vi "Detect Modules.vi"(8 "error in":errorcluster, 9 "Chassis in":refnum<class "Chassis.lvclass">, 10 "Controller in":refnum<class "Controller.lvclass">, 11 "Device in":refnum<class "SysCfg Device.lvclass">) -> (0 "error out":errorcluster, 1 "Chassis out":refnum<class "Chassis.lvclass">, 2 "Controller out":refnum<class "Controller.lvclass">, 3 "Device out":refnum<class "SysCfg Device.lvclass">)   [LabVIEW 2015, in "SMI.lvlib" / "Chassis.lvclass"]
uses:
  Chassis.lvclass
  SysCfg Device/SysCfg Device.lvclass
  Controller/Controller.lvclass
  Device/Device.lvclass/Device.ctl
  Chassis.lvclass/Chassis.ctl
  Module/Module.lvclass
  Device/Accessor Methods/Read Product Name.vi
  <vilib>/FPGAPlugInAG/Dynamic/niLvFpga_Close_Dynamic.vi
  <vilib>/regexp/Match Regular Expression.xnode
  <vilib>/rvi/interface/nirviCloseFPGA/nirviCloseFPGA.xnode
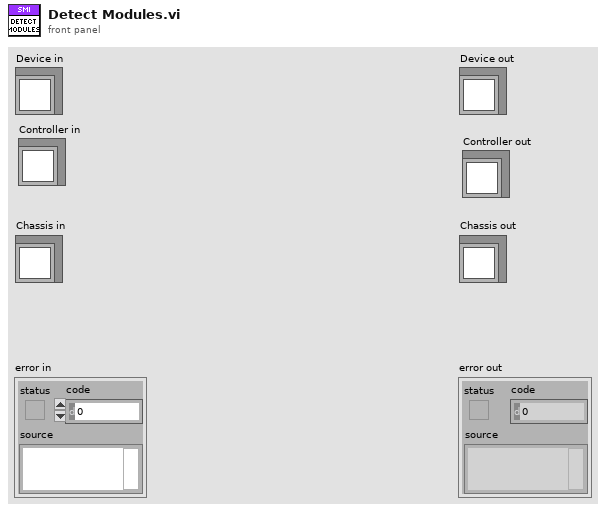
[diagram p1: front panel]
types:
  T1 = typedef "SMI.lvlib/Module.lvclass/ModuleInformation.ctl" = cluster{"Vendor":string, "Model":string, "Module Code":u32, "Serial Number":string}
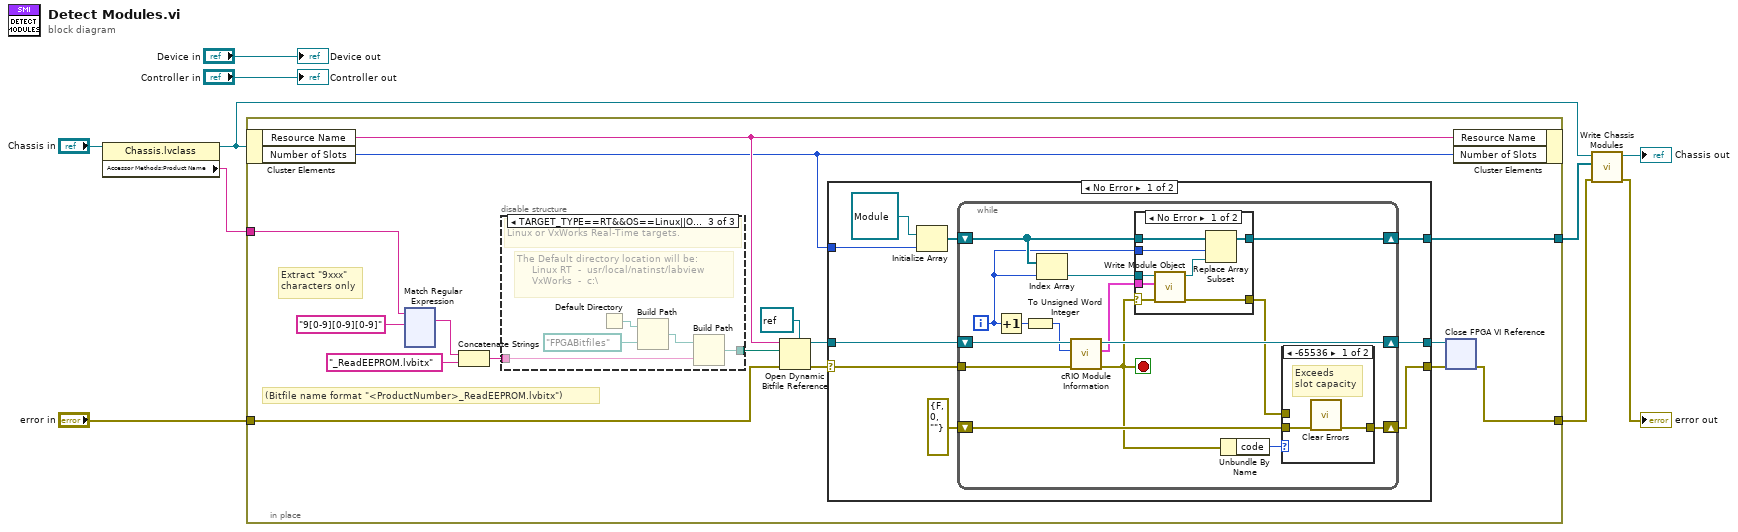
[diagram p0: block diagram]
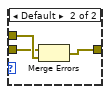
[diagram p2: hidden frame]
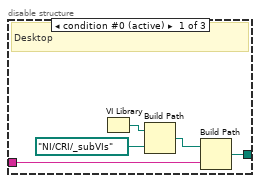
[diagram p5: hidden frame]
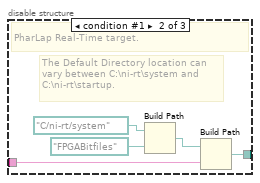
[diagram p6: hidden frame]
diagram:
  n1 = property class="Chassis.lvclass"(reference="Chassis in") -> (reference out=w2:refnum<class "Chassis.lvclass">, "Accessor Methods:Product Name"=w1:string)  [unwired: 1 in, 1 out]
  n2 = in-place {
    in-place-border: "error in" -> [w18]
    in-place-border: [w14] -> w5
    in-place-border: [w13] -> w4
    in-place-border: w1 -> [w11]
    # "Extract \"9xxx\"\ncharacters only"
    # "(Bitfile name format \"<ProductNumber>_ReadEEPROM.lvbitx\")"
    n3 = in-place-cluster #1(w2) -> ("Resource Name"=w17:string, "Number of Slots"=w12:i32)
    n4 = xnode "Match Regular Expression"("input string"=w11, "regular expression"="9[0-9][0-9][0-9]") -> ("whole match"=w25:string)  [unwired: 4 in, 4 out]
    n5 = Concatenate Strings(w25, "_ReadEEPROM.lvbitx" ("string")) -> (w23:string)
    n6 = disable-structure shown="TARGET_TYPE==RT&&OS==Linux||OS==VxWorks" {
      disable-tunnel: w23 -> [w72 w77 w82]
      disable-tunnel: [w71 w76 w81] -> w19
      frame condition #0 (active) {
        # "Desktop"
        n7 = VI Library() -> (path=w70:path)
        n8 = Build Path(base path=w70, name or relative path=path "NI/CRI/_subVIs") -> (appended path=w68:path)
        n9 = Build Path(base path=w68, name or relative path=w72) -> (appended path=w71:path)
      }
      frame condition #1 {
        # "The Default Directory location can\nvary between C:\\ni-rt\\system and\nC:\\ni-rt\\startup."
        # "PharLap Real-Time target."
        n10 = Build Path(base path=path "C:/ni-rt/system", name or relative path=path "FPGABitfiles") -> (appended path=w75:path)
        n11 = Build Path(base path=w75, name or relative path=w77) -> (appended path=w76:path)
      }
      frame condition #2 {
        # "The Default directory location will be:\n     Linux RT  -  usr/local/natinst/labview\n     VxWorks  -  c:\\"
        # "Linux or VxWorks Real-Time targets."
        n12 = Default Directory() -> (w78:path)
        n13 = Build Path(base path=w78, name or relative path=path "FPGABitfiles") -> (appended path=w80:path)
        n14 = Build Path(base path=w80, name or relative path=w82) -> (appended path=w81:path)
      }
    }
    n15 = Open Dynamic Bitfile Reference(0:w17, 1:w19, 3:w18, 4:refnum<k20> refnum ("Refnum out")) -> (5:w21:refnum<k20>, 8:w22:errorcluster)  [unwired: 1 in]
    n16 = case shown="No Error" w22 {
      selector: w22 -> [w34 w67]
      tunnel: w21 -> [w35 w66]
      tunnel: [w33 _] -> w13
      tunnel: [w32 w66] -> w16
      tunnel: [w31 w67] -> w15
      tunnel: w12 -> [w27 _]
      frame No Error {
        n17 = Initialize Array(refnum<class "Module.lvclass"> refnum ("RT Management.lvlib:Module Detection.lvclass"), w27) -> (w28:refnum<class "Module.lvclass">[])
        n18 = while {
          shift-right: [w48] -> w32
          shift-left: w35 -> [w50]
          tunnel: w34 -> [w49]
          shift-right: [w44] -> w33
          shift-left: w28 -> [w43]
          shift-right: [w38] -> w31
          shift-left: errorcluster {"status"=FALSE, "code"=0, "source"=""} ("error IO") -> [w39]
          i -> [w41]
          stop <- w37 stop-if-true
          n19 = Increment(x=w41) -> (x+1=w47:i32)
          n20 = To Unsigned Word Integer(number=w47) -> (unsigned 16bit integer=w46:u16)
          n21 = Index Array(array=w43, index=w41) -> (element=w42:refnum<class "Module.lvclass">)
          n22 = call "cRIO Module Information.vi"("error in"=w49, "Module"=w46, "Refnum in"=w50) -> ("error out"=w37:errorcluster, "cRIO Module Information"=w45:T1, "Refnum out"=w48:refnum<k20>)  [unwired: 6 in]
          n23 = case shown="No Error" w37 {
            selector: w37 -> [w57 w64]
            tunnel: w45 -> [w63 _]
            tunnel: [w62 w65] -> w44
            tunnel: w43 -> [w60 w65]
            tunnel: w42 -> [w59 _]
            tunnel: w41 -> [w58 _]
            tunnel: [w56 w64] -> w40
            frame No Error {
              n24 = call "Write Module Object.vi"("error in"=w57, "Module Information"=w63, "Module Detection in"=w59) -> ("error out"=w56:errorcluster, "Module Detection out"=w61:refnum<class "Module.lvclass">)  [unwired: 7 in]
              n25 = Replace Array Subset(array=w60, new element=w61, index=w58) -> (w62:refnum<class "Module.lvclass">[])
            }
            frame Error {
            }
          }
          n26 = Unbundle By Name(w37) -> ("code"=w36:i32)
          n27 = case shown="-65536" w36 {
            tunnel: w40 -> [_ w55]
            tunnel: w39 -> [w52 w54]
            tunnel: [w51 w53] -> w38
            frame -65536 {
              # "Exceeds\nslot capacity"
              n28 = call <vilib>:"Clear Errors.vi"("error in (no error)"=w52) -> ("error out"=w51:errorcluster)  [unwired: 5 in, 1 out]
            }
            frame Default {
              n29 = Merge Errors(w54, w55) -> (w53:errorcluster)
            }
          }
        }
      }
      frame Error {
      }
    }
    n30 = xnode "Close FPGA VI Reference"("FPGA VI Reference In"=w16, "error in"=w15) -> ("error out"=w14:errorcluster)
    n31 = in-place-cluster #1("Resource Name"=w17, "Number of Slots"=w12) -> ()  [unwired: 1 out]
  }
  n32 = call "Write Chassis Modules.vi"("error in"=w5, "Modules"=w4, "Chassis in"=w2) -> ("error out"=→"error out":errorcluster, "Chassis out"=→"Chassis out":refnum<class "Chassis.lvclass">)  [unwired: 7 in]
  "Device out" <- "Device in"
  "Controller out" <- "Controller in"
